vi "Joystick Control to Command.vi"(11 "Robot Controls":T2) -> (3 "Robot Commands":T1)   [LabVIEW 2014]
uses:
  Robot Controls.ctl
  Robot Commands.ctl
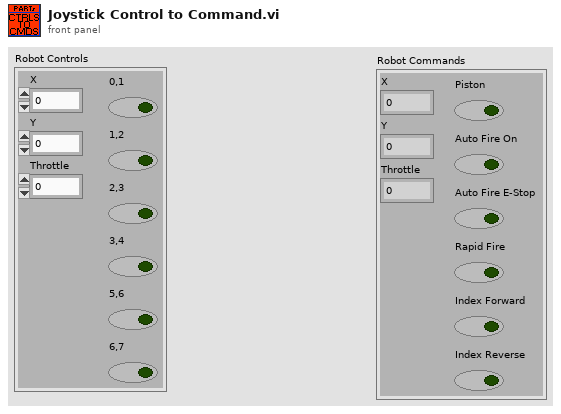
[diagram p1: front panel]
types:
  T1 = typedef "Robot Commands.ctl" = cluster{"X":dbl, "Y ":dbl, "Throttle":dbl, "Piston":bool, "Auto Fire On":bool, "Auto Fire E-Stop":bool, "Rapid Fire":bool, "Index Forward":bool, "Index Reverse ":bool}
  T2 = typedef "Robot Controls.ctl" = cluster{"X":dbl, "Y ":dbl, "Throttle":dbl, "0,1":bool, "1,2":bool, "2,3":bool, "3,4":bool, "5,6":bool, "6,7 ":bool}
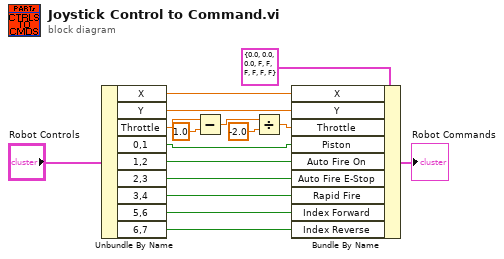
[diagram p0: block diagram]
diagram:
  n1 = Unbundle By Name("Robot Controls") -> ("X"=w11:dbl, "Y"=w10:dbl, "Throttle"=w12:dbl, "0,1"=w8:bool, "1,2"=w7:bool, "2,3"=w6:bool, "3,4"=w3:bool, "5,6"=w2:bool, "6,7"=w1:bool)
  n2 = Subtract(x=w12, y=1.0) -> (x-y=w13:dbl)
  n3 = Divide(x=w13, y=-2.0) -> (x/y=w9:dbl)
  n4 = Bundle By Name(cluster=T1 {"X"=0.0, "Y "=0.0, "Throttle"=0.0, "Piston"=FALSE, "Auto Fire On"=FALSE, "Auto Fire E-Stop"=FALSE, "Rapid Fire"=FALSE, "Index Forward"=FALSE, "Index Reverse "=FALSE} ("Robot Comands"), "X"=w11, "Y"=w10, "Throttle"=w9, "Piston"=w8, "Auto Fire On"=w7, "Auto Fire E-Stop"=w6, "Rapid Fire"=w3, "Index Forward"=w2, "Index Reverse"=w1) -> (→"Robot Commands":T1)
